vi "Modbus Multi-Write U16.vi"(7 "Slave Address":u8, 8 "error in (no error)":errorcluster, 9 "Input data [U16]":u16[](array[numeric]), 10 "Register Start Address":u16 format="%x", 11 "VISA resource in":refnum<visa-resource-name>) -> (0 "error out":errorcluster, 3 "VISA resource out":refnum<visa-resource-name>)   [LabVIEW 2010, in "Voegtlin_NI_SMART_Modbus_Drivers.lvlib"]
doc: "Schreibe die uebergebene Anzahl U16-Werte an die angegebene Startadresse des selektierten Geraetes.\nDer COM-Port muss dazu initialisiert sein (benutze\" Modbus Init.vi\")."
uses:
  Voegtlin_NI_SMART_Modbus_Drivers.lvlib
  Enums/Modbus Comm.ctl
panel:
  # "Input Data"
  # "Internal Data"
  # "Output Data"
  # "(Inputmaske in HEX)"
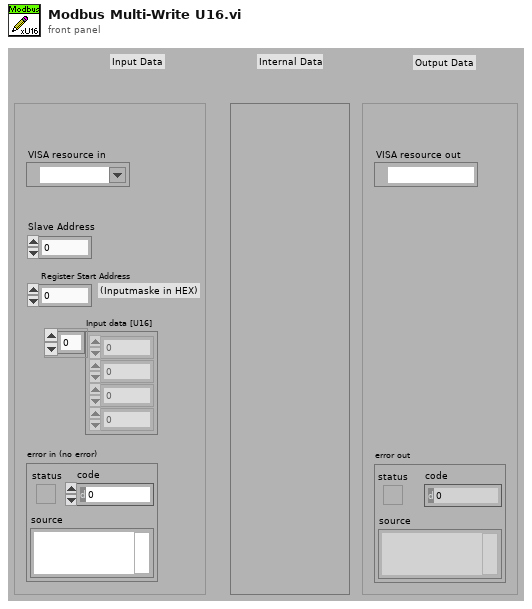
[diagram p1: front panel]
types:
  T1 = typedef "Voegtlin_NI_SMART_Modbus_Drivers.lvlib/Modbus Comm.ctl" = enum16{"Init", "Read", "Write", "Exit"}
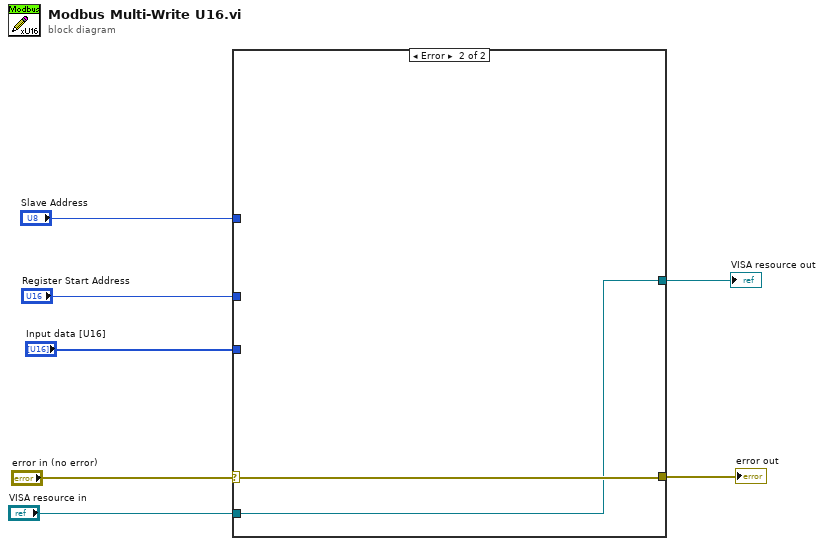
[diagram p0: block diagram]
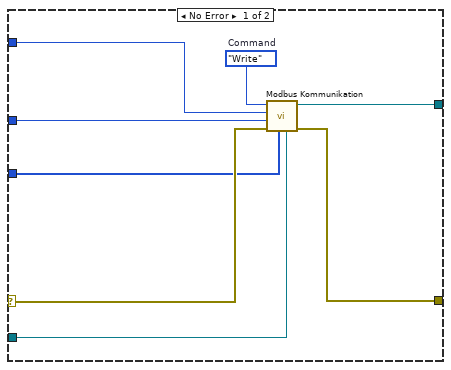
[diagram p2: hidden frame]
diagram:
  n1 = case shown="Error" "error in (no error)" {
    selector: "error in (no error)" -> [w13 w17]
    tunnel: "Register Start Address" -> [w11 _]
    tunnel: [w15 w17] -> w6
    tunnel: "Input data [U16]" -> [w12 _]
    tunnel: "Slave Address" -> [w10 _]
    tunnel: "VISA resource in" -> [w9 w16]
    tunnel: [w8 w16] -> w1
    frame No Error {
      w14 = Modbus_Comm."Write"  # Command
      n2 = call "Modbus Kommunikation.vi"("VISA resource in"=w9, "Data In / #Reads [U16]"=w12, "error in (no error)"=w13, "Register Start Address"=w11, "Slave Address"=w10, "Command"=w14) -> ("error out"=w15:errorcluster, "VISA resource out"=w8:refnum<visa-resource-name>)  [unwired: 3 in, 1 out]
    }
    frame Error {
    }
  }
  "error out" <- w6
  "VISA resource out" <- w1
